vi "hidSPD List Devices.vi"(8 "error in (no error)":errorcluster) -> (0 "error out":errorcluster, 2 "devices list":T1[](array[typedef]))   [LabVIEW 2018, in "hidSPDLibForLabView.lvlib"]
uses:
  hidSPDLibForLabView.lvlib
  hidSPD Controls/hidSPD HidDevInfo.ctl
  hidSPD DLL files/libSPD.dll
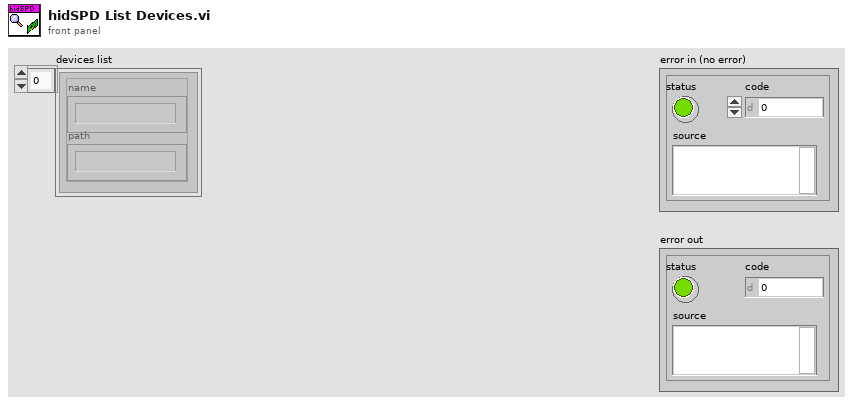
[diagram p1: front panel]
types:
  T1 = typedef "hidSPDLibForLabView.lvlib/hidSPD HidDevInfo.ctl" = cluster{"name":string, "path":string}
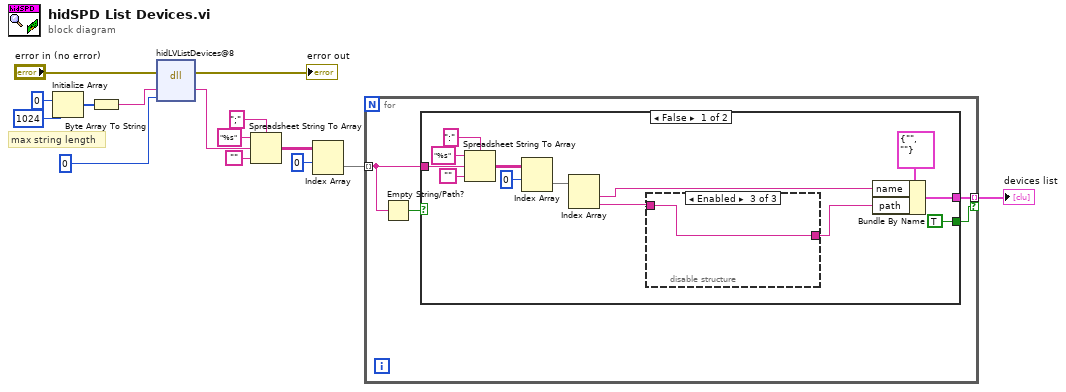
[diagram p0: block diagram]
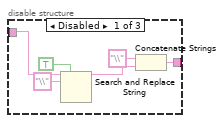
[diagram p2: hidden frame]
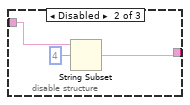
[diagram p3: hidden frame]
diagram:
  # "max string length"
  n1 = Initialize Array(u8 0 ("element"), 1024 ("dimension size")) -> (w10:u8[])
  n2 = Byte Array To String(unsigned byte array=w10) -> (string=w9:string)
  n3 = dll-call lib="D:/NextCloud/SPD/hidSPDLibForLabView/hidSPD DLL files/libSPD.dll" fn="hidLVListDevices@8"(error in="error in (no error)", "spdDevList"=w9, "listLength"=0) -> (error out=→"error out":errorcluster, "spdDevList"=w2:string)  [unwired: 4 in, 1 out]
  n4 = Spreadsheet String To Array(delimiter (Tab)=";", format string="%s", spreadsheet string=w2, array type (2D Dbl)="") -> (array=w5:string[][])
  n5 = Index Array(array=w5, index (row)=0) -> (element=w3:string[])  [unwired: 1 in]
  n6 = for {
    tunnel: w3 -> [w17] mode=indexing
    tunnel: [w19] -> w1 mode=indexing if=w16
    n7 = Empty String/Path?(string/path=w17) -> (empty?=w18:bool)
    n8 = case shown="False" w18 {
      tunnel: w17 -> [w29 _]
      tunnel: [w23 _] -> w19
      tunnel: [TRUE _] -> w16
      frame False {
        n9 = Spreadsheet String To Array(delimiter (Tab)=":", format string="%s", spreadsheet string=w29, array type (2D Dbl)="") -> (array=w28:string[][])
        n10 = Index Array(array=w28, index (row)=0) -> (element=w26:string[])  [unwired: 1 in]
        n11 = Index Array(array=w26) -> (element #1=w24:string, element #2=w21:string)  [unwired: 2 in]
        n12 = disable-structure shown="Enabled" {
          disable-tunnel: w21 -> [w38 w41 w42]
          disable-tunnel: [w33 w39 w42] -> w20
          frame Disabled {
            n13 = Search and Replace String(replace all?=TRUE ("replace all? (F)"), input string=w38, search string="\\") -> (result string=w35:string)  [unwired: 5 in, 3 out]
            n14 = Concatenate Strings("\\" ("string"), w35) -> (w33:string)
          }
          frame Disabled {
            n15 = String Subset(string=w41, offset (0)=4) -> (substring=w39:string)  [unwired: 1 in]
          }
          frame Enabled {
          }
        }
        n16 = Bundle By Name(cluster=T1 {"name"="", "path"=""} ("HidDevInfo"), "name"=w24, "path"=w20) -> (w23:T1)
      }
      frame True {
      }
    }
  }
  "devices list" <- w1
